vi "Calibrate Using the NI Calibration Dot Matrix.vi"(11 "Camera Name":string) -> (0 "error out":errorcluster, 3 "Insufficient Data":bool)   [LabVIEW 2025]
uses:
  <vilib>/Utility/sysdir.llb/System Directory Type.ctl
  <vilib>/vision/NI_Vision_Development_Module.lvlib
panel:
  out "Dots matrix":T1(plugin-control)
  out "Original":T1(plugin-control)
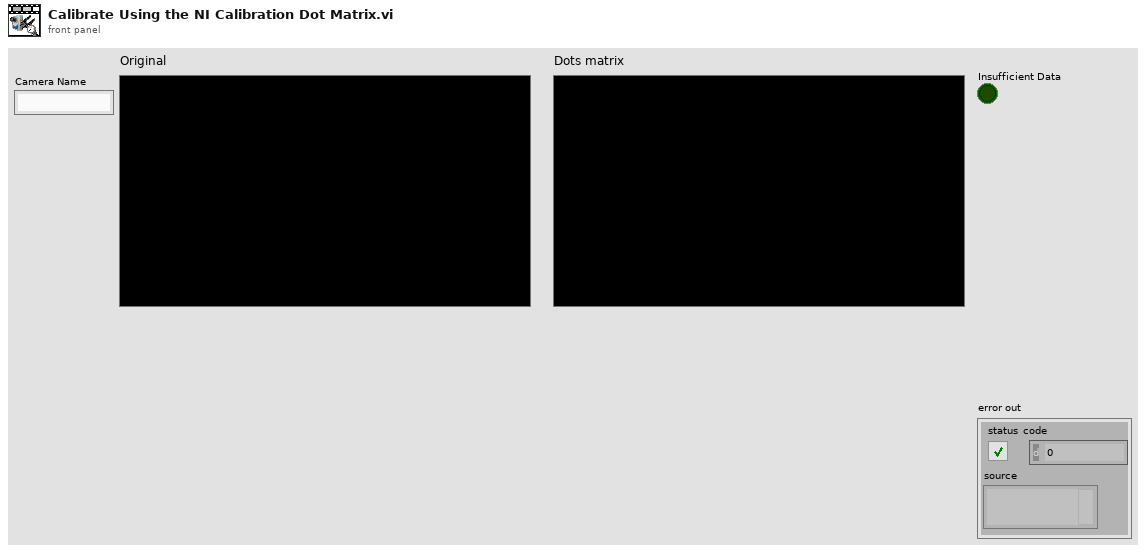
[diagram p1: front panel]
types:
  T1 = typedef "IMAQ Image.ctl" = refnum<image>
  T2 = typedef "System Directory Type.ctl" = i32
  T3 = typedef "Image Unit" = enum32{"Undefined", "Angström", "Micrometer", "Millimeter", "Centimeter", "Meter", "Kilometer", "Microinch", "Inch", "Feet", "Nautical miles", "Standard miles", "Steps"}
  T4 = typedef "Particle Parameters" = i32
  T5 = cluster{"Measurement Parameter":T4, "Range Lower Value":dbl, "Range Upper Value":dbl, "Range":bool, "Measurement Type":bool}[]
  T6 = typedef "Image Type" = u32
  T7 = typedef "Calibration Reference Points.ctl" = cluster{"Pixel Coordinates":cluster{"X":dbl, "Y":dbl}[], "Real World Coordinates":cluster{"X":dbl, "Y":dbl}[], "Unit":T3, "Image Size":cluster{"X":u32, "Y":u32}}
  T8 = typedef "Internal Parameters.ctl" = cluster{"Insufficient Data":bool, "Focal Length (pixel)":cluster{"fx":sgl, "fy":sgl}, "Optical Center (pixel)":cluster{"cx":sgl, "cy":sgl}}
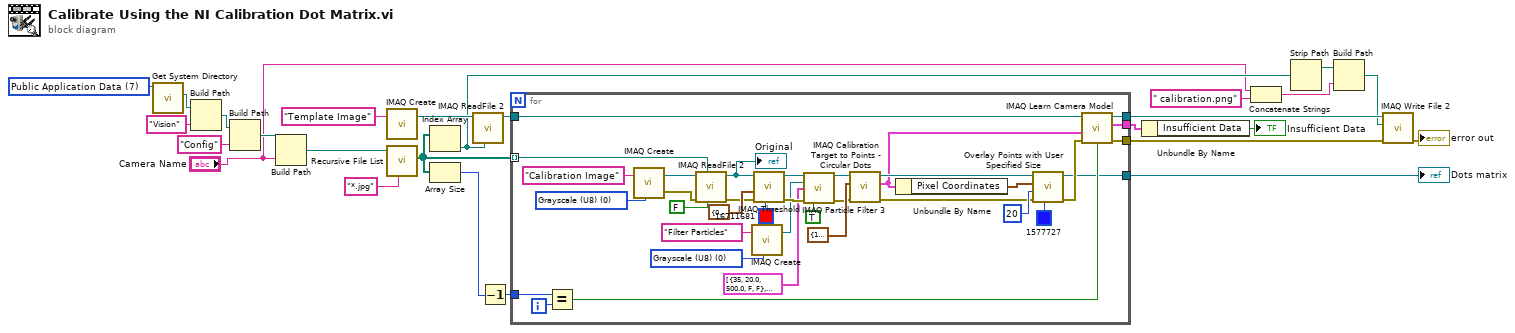
[diagram p0: block diagram]
diagram:
  w11 = T2 7 items=["User Home"=0, "User Desktop"=1, "User Documents"=2, "User Application Data"=3, "User Preferences"=4, "User Temporary"=5, "Public Documents"=6, "Public Application Data"=7, "Public Preferences"=8, "Public Cache"=13, "System Core Libraries"=9, "System Installed Libraries"=10, "Application Files"=11, "Boot Volume Root"=12] ("system directory type")
  n1 = call <vilib>:"Get System Directory.vi"("system directory type"=w11) -> ("system directory"=w8:path)  [unwired: 10 in]
  n2 = Build Path(base path=w8, name or relative path="Vision") -> (appended path=w9:path)
  n3 = Build Path(base path=w9, name or relative path="Config") -> (appended path=w7:path)
  n4 = Build Path(base path=w7, name or relative path="Camera Name") -> (appended path=w6:path)
  n5 = call "IMAQ Create"("Image Name"="Template Image") -> ("New Image"=w21:T1)  [unwired: 4 in, 1 out]
  n6 = call <vilib>:"Recursive File List.vi"("pattern"="*.jpg", "Folder Path"=w6) -> ("All Files in Dir"=w23:path[])  [unwired: 5 in, 4 out]
  n7 = Index Array(array=w23) -> (element=w17:path)  [unwired: 1 in]
  n8 = Array Size(array=w23) -> (size(s)=w24:i32)
  n9 = call "IMAQ ReadFile 2"("File Path"=w17, "Image"=w21) -> ("Image Out"=w20:T1)  [unwired: 5 in, 4 out]
  n10 = Decrement(x=w24) -> (x-1=w25:i32)
  n11 = for {
    tunnel: w23 -> [w42] mode=indexing
    tunnel: w25 -> [w37]
    tunnel: [w33] -> w13
    tunnel: [w32] -> w19
    tunnel: w20 -> [w31]
    tunnel: [w30] -> w18
    tunnel: [w29] -> w2
    i -> [w38]
    w50 = T6 0 items=["Grayscale (U8)", "Grayscale (I16)", "Grayscale (SGL)", "Complex (CSG)", "RGB (U32)", "HSL (U32)", "RGB (U64)", "Grayscale (U16)"] ("Image Type")
    w61 = T6 0 items=["Grayscale (U8)", "Grayscale (I16)", "Grayscale (SGL)", "Complex (CSG)", "RGB (U32)", "HSL (U32)", "RGB (U64)", "Grayscale (U16)"] ("Image Type")
    n12 = Equal?(x=w37, y=w38) -> (x = y?=w36:bool)
    n13 = call "IMAQ Create"("Image Name"="Calibration Image", "Image Type"=w61) -> ("New Image"=w59:T1, "error out"=w58:errorcluster)  [unwired: 3 in]
    n14 = call "IMAQ ReadFile 2"("Use File Path Image Type"=FALSE, "File Path"=w42, "error in (no error)"=w58, "Image"=w59) -> ("error out"=w56:errorcluster, "Image Out"=w45:T1)  [unwired: 3 in, 3 out]
    "Original" <- w45
    n15 = call "IMAQ Create"("Image Name"="Filter Particles", "Image Type"=w50) -> ("New Image"=w49:T1)  [unwired: 3 in, 1 out]
    n16 = call "IMAQ Threshold"("Replace Value"=u32 16711681 ("Color"), "error in (no error)"=w56, "Range"=cluster{"Lower value":sgl, "Upper value":sgl} {"Lower value"=0.0, "Upper value"=60.0}, "Image Src"=w45) -> ("error out"=w54:errorcluster, "Image Dst Out"=w44:T1)  [unwired: 6 in]
    n17 = call "IMAQ Particle Filter 3"("Image Src"=w44, "Image Dst"=w49, "Selection Values"=T5 [{"Measurement Parameter"=35, "Range Lower Value"=20.0, "Range Upper Value"=500.0, "Range"=FALSE, "Measurement Type"=FALSE}, {"Measurement Parameter"=55, "Range Lower Value"=0.8, "Range Upper Value"=1.2, "Range"=FALSE, "Measurement Type"=FALSE}], "error in (no error)"=w54, "Reject Border? (F)"=TRUE) -> ("Image Dst Out"=w43:T1, "error out"=w41:errorcluster)  [unwired: 8 in, 1 out]
    n18 = call "IMAQ Calibration Target to Points - Circular Dots"("error in (no error)"=w41, "Grid Descriptor"=cluster{"X Step":sgl, "Y Step":sgl, "Unit":T3} {"X Step"=1.0, "Y Step"=1.0, "Unit"=enum."Centimeter"}, "Target Image"=w43) -> ("error out"=w40:errorcluster, "Reference Points"=w27:T7, "Target Image (dup)"=w39:T1)  [unwired: 2 in, 4 out]
    n19 = Unbundle By Name(w27) -> ("Pixel Coordinates"=w47:cluster{"X":dbl, "Y":dbl}[])
    n20 = call "Overlay Points with User Specified Size.vi"("Color"=u32 1577727, "error in"=w40, "Point Diameter (5)"=u32 20 ("Point Size (5)"), "Points"=w47, "Image In"=w39) -> ("error out"=w35:errorcluster, "Image Out"=w32:T1)  [unwired: 5 in]
    n21 = call "IMAQ Learn Camera Model"("Add Points and Learn (True)"=w36, "error in (no error)"=w35, "Reference Points"=w27, "Calibration Template Image"=w31) -> ("error out"=w33:errorcluster, "Internal Parameters"=w29:T8, "Calibration Template Image Out"=w30:T1)  [unwired: 5 in]
  }
  "Dots matrix" <- w19
  n22 = Unbundle By Name(w2) -> ("Insufficient Data"=→"Insufficient Data":bool)
  n23 = Concatenate Strings("Camera Name", " calibration.png" ("string")) -> (w5:string)
  n24 = Strip Path(path=w17) -> (stripped path=w15:path)  [unwired: 1 out]
  n25 = Build Path(base path=w15, name or relative path=w5) -> (appended path=w14:path)
  n26 = call-poly "IMAQ Write File 2"("error in (no error)"=w13, "File Path"=w14, "Image"=w18) -> ("error out"=→"error out":errorcluster)  [unwired: 7 in, 1 out]
